vi "PWM Control.vi"() -> ()   [LabVIEW 2019]
uses:
  <vilib>/MakerHub/LINX/Public/Utilities/Open Serial.vi
  <vilib>/MakerHub/LINX/Public/Sensors/Motion/Servo/Servo Open One Channel.vi
  <vilib>/MakerHub/LINX/Public/Sensors/Motion/Servo/Servo Set Pulse Width One Channel.vi
  <vilib>/MakerHub/LINX/Public/Sensors/Motion/Servo/Servo Close One Channel.vi
  <vilib>/MakerHub/LINX/LMH-LINX.lvlib
  <vilib>/MakerHub/LINX/Public/Sensors/Motion/Servo/Servo.lvlib
panel:
  in  "Serial Port":refnum<visa-resource-name>="N/A"
  in  "Pulse Width (uS)":u16(knob) scale=0.0..2000.0
  in  "Servo Channel":u8
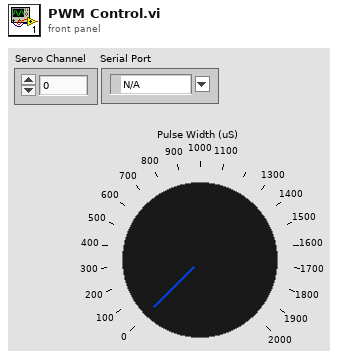
[diagram p1: front panel]
types:
  T1 = typedef "LMH-LINX.lvlib/LINX Ref.ctl" = cluster{"IO":T2, "Interface":T3, "LINX Device Config":T4}
  T2 = typedef "LMH-LINX.lvlib/Platform.ctl" = enum16{"Remote", "Local"}
  T3 = typedef "LMH-LINX.lvlib/Interface.ctl" = enum16{"Serial", "TCP"}
  T4 = typedef "LMH-LINX.lvlib/Device.lvlib/LINX Device Config.ctl" = cluster{"Interface":T3, "COM Port":refnum<visa-resource-name>, "TCP Configuration":T5, "Device Family":u8, "Device ID":u8, "Device Name":string, "TCP Ref":refnum<k5>, "Channels":T6}
  T5 = typedef "LMH-LINX.lvlib/Device.lvlib/TCP Config.ctl" = cluster{"IP Address":string, "Port":u16}
  T6 = typedef "LMH-LINX.lvlib/Channels.ctl" = cluster{"DI":u8[], "DO":u8[], "AI":u8[], "AO":u8[], "PWM":u8[], "QE":u8[], "UART":u8[], "I2C 2":u8[], "SPI":u8[], "CAN":u8[], "Servo":u8[], "AI Ref (V)":dbl, "AI Resolution (Bits)":u8, "AO Ref (V)":dbl, "AO Resolution (Bits)":u8}
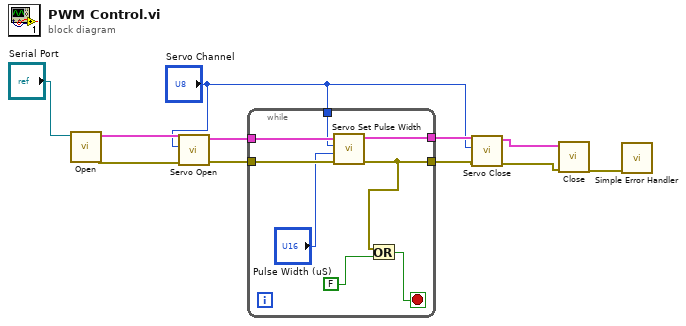
[diagram p0: block diagram]
diagram:
  n1 = call-poly <vilib>:"Open.vi"("Serial Port"="Serial Port") -> ("Error Out"=w8:errorcluster, "LINX Resource"=w7:T1)  [unwired: 8 in, 1 out]
  n2 = call-poly <vilib>:"Servo Open.vi"("Error In"=w8, "Servo Channel"="Servo Channel", "LINX Resource"=w7) -> ("Error Out"=w9:errorcluster, "LINX Resource"=w6:T1)  [unwired: 7 in]
  n3 = while {
    tunnel: [w17] -> w11
    tunnel: w9 -> [w16]
    tunnel: w6 -> [w15]
    tunnel: [w14] -> w5
    tunnel: "Servo Channel" -> [w13]
    stop <- w19 stop-if-true
    n4 = call-poly <vilib>:"Servo Set Pulse Width.vi"("Error In"=w16, "Pulse Width (uS)"="Pulse Width (uS)", "Servo Channel"=w13, "LINX Resource"=w15) -> ("Error Out"=w17:errorcluster, "LINX Resource"=w14:T1)  [unwired: 6 in]
    n5 = Or(x=w17, y=FALSE ("stop")) -> (x .or. y?=w19:bool)
  }
  n6 = call-poly <vilib>:"Servo Close.vi"("Error In"=w11, "Servo Channel"="Servo Channel", "LINX Resource"=w5) -> ("Error Out"=w10:errorcluster, "LINX Resource"=w4:T1)  [unwired: 7 in]
  n7 = call <vilib>:"Close.vi"("Error In"=w10, "LINX Resource"=w4) -> ("Error Out"=w1:errorcluster)  [unwired: 9 in]
  n8 = call <vilib>:"Simple Error Handler.vi"("error in (no error)"=w1) -> ()  [unwired: 4 in, 5 out]
